vi "Sub_FEA_Make_M_and K_Matrices_preloop.vi"(11 "Setup Parameters":T1) -> (3 "FEA matrices":cluster{"Mass":dbl[][], "Stiffness":dbl[][]})   [LabVIEW 2019]
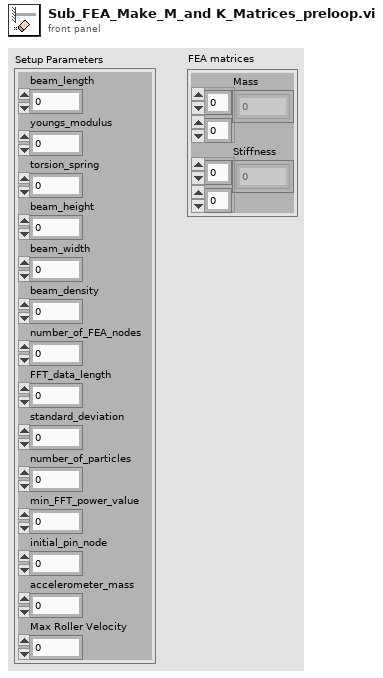
[diagram p1: front panel]
types:
  T1 = cluster{"beam_length":dbl, "youngs_modulus":dbl, "torsion_spring":dbl, "beam_height":dbl, "beam_width":dbl, "beam_density":dbl, "number_of_FEA_nodes":i32, "FFT_data_length":i32, "standard_deviation":dbl, "number_of_particles":i32, "min_FFT_power_value":dbl, "initial_pin_node":i32, "accelerometer_mass":dbl, "Max Roller Velocity":dbl}
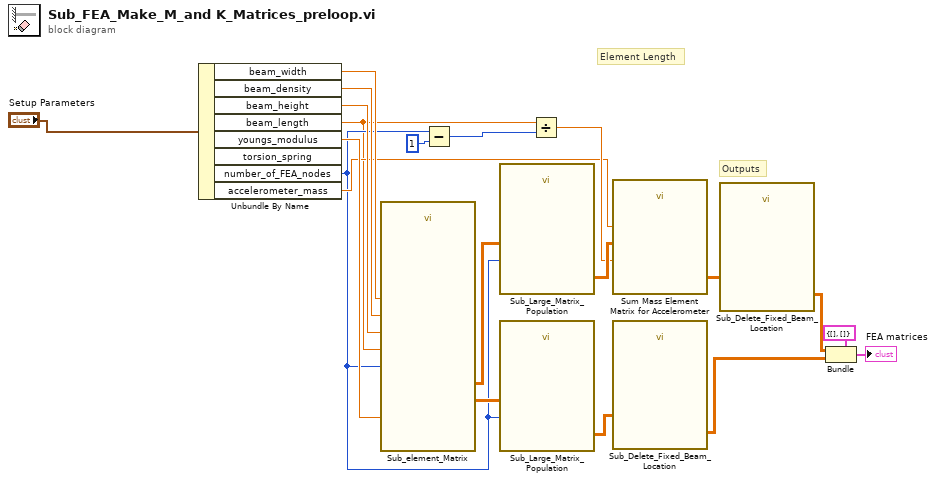
[diagram p0: block diagram]
diagram:
  # "Outputs"
  # "Element Length"
  n1 = Unbundle By Name("Setup Parameters") -> ("beam_width"=w14:dbl, "beam_density"=w15:dbl, "beam_height"=w16:dbl, "beam_length"=w6:dbl, "youngs_modulus"=w17:dbl, "number_of_FEA_nodes"=w7:i32, "accelerometer_mass"=w8:dbl)  [unwired: 1 out]
  n2 = call "Sub_element_Matrix.vi"("Length of Beam"=w6, "Young's Modulus"=w17, "No. of Nodes"=w7, "Height"=w16, "Width"=w14, "Density"=w15) -> ("M Element Matrix"=w18:dbl[][], "K Element Matrix"=w19:dbl[][])  [unwired: 11 in, 1 out]
  n3 = Subtract(x=w7, y=1) -> (x-y=w11:i32)
  n4 = call "Sub_Large_Matrix_Population.vi"("No. of Nodes"=w7, "Element Matrix"=w18) -> ("Matrix w/o BC"=w12:dbl[][])  [unwired: 9 in]
  n5 = call "Sub_Large_Matrix_Population.vi"("No. of Nodes"=w7, "Element Matrix"=w19) -> ("Matrix w/o BC"=w20:dbl[][])  [unwired: 9 in]
  n6 = Divide(x=w6, y=w11) -> (x/y=w9:dbl)
  n7 = call "Sum Mass Element Matrix for Accelerometer.vi"("Matrix w/o BC"=w12, "accelerometer_mass"=w8, "Element Length"=w9) -> ("Matrix W/ Accelerometer"=w13:dbl[][])  [unwired: 8 in]
  n8 = call "Sub_Delete_Fixed_Beam_Location.vi"("Pre-BC Matrix"=w20) -> ("Post-BC Matrix"=w1:dbl[][])  [unwired: 10 in]
  n9 = call "Sub_Delete_Fixed_Beam_Location.vi"("Pre-BC Matrix"=w13) -> ("Post-BC Matrix"=w2:dbl[][])  [unwired: 10 in]
  n10 = Bundle(cluster=cluster{"Mass":dbl[][], "Stiffness":dbl[][]} {"Mass"=[], "Stiffness"=[]} ("FEA matrices"), "Mass"=w2, "Stiffness"=w1) -> (→"FEA matrices":cluster{"Mass":dbl[][], "Stiffness":dbl[][]})
